vi "get_command_position.vi"(8 "error in (no error)":errorcluster, 11 "DL090409StageScaffold.lvclass in":refnum<class "StageDL090409Scaffold.lvclass">) -> (0 "error out":errorcluster, 2 "SpaceVector.lvclass":refnum<class "SpaceVector.lvclass">, 3 "DL090409StageScaffold.lvclass out":refnum<class "StageDL090409Scaffold.lvclass">)   [LabVIEW 2010, in "StageDL090409Scaffold.lvclass"]
uses:
  StageDL090409Scaffold.lvclass
  common/classes/SpaceVector/SpaceVector/SpaceVector.lvclass
  StageDL090409Scaffold.lvclass/StageDL090409Scaffold.ctl
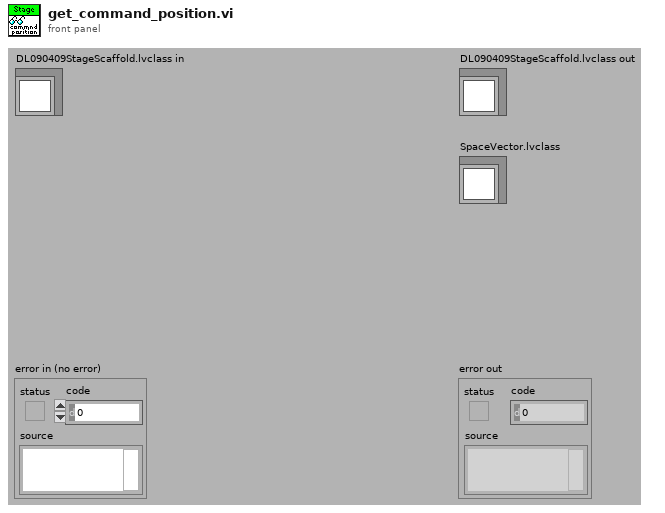
[diagram p1: front panel]
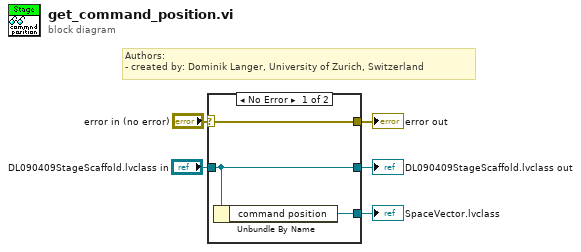
[diagram p0: block diagram]
diagram:
  # "Authors: \n- created by: Dominik Langer, University of Zurich, Switzerland"
  n1 = case shown="No Error" "error in (no error)" {
    selector: "error in (no error)" -> [w8 w9]
    tunnel: [w8 w9] -> w4
    tunnel: [w7 w10] -> w2
    tunnel: "DL090409StageScaffold.lvclass in" -> [w7 w10]
    tunnel: [w6 _] -> w1
    frame No Error {
      n2 = Unbundle By Name(w7) -> ("command position"=w6:refnum<class "SpaceVector.lvclass">)
    }
    frame Error {
    }
  }
  "error out" <- w4
  "DL090409StageScaffold.lvclass out" <- w2
  "SpaceVector.lvclass" <- w1
